vi "WriteFiles.vi"(8 "error in (no error)":errorcluster caption="错误输入（无错误）", 11 "EPUB 输入":refnum<class "EPUB.lvclass">) -> (0 "error out":errorcluster caption="错误输出", 3 "EPUB 输出":refnum<class "EPUB.lvclass">)   [LabVIEW 2016, in "EPUB.lvclass"]
uses:
  EPUB.lvclass
  EPUB.lvclass/EPUB.ctl
  <vilib>/NUAA/UTF8Convert.llb/Text2UTF8.vi
  <vilib>/Utility/libraryn.llb/Get File Extension.vi
  <userlib>/_OpenG.lib/string/string.llb/1D Array to String__ogtk.vi
  IMGSettings.vi
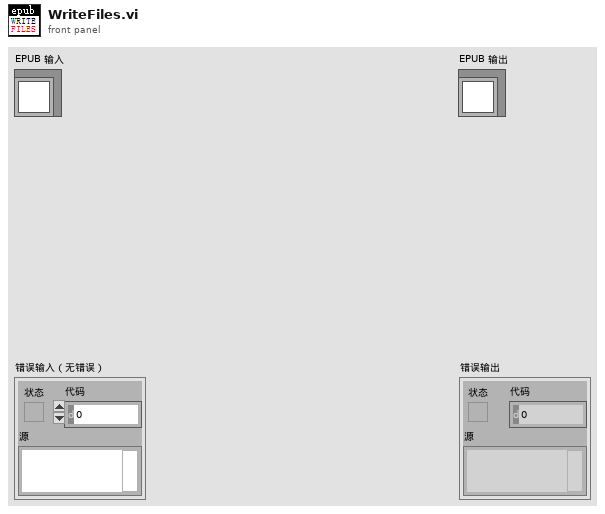
[diagram p1: front panel]
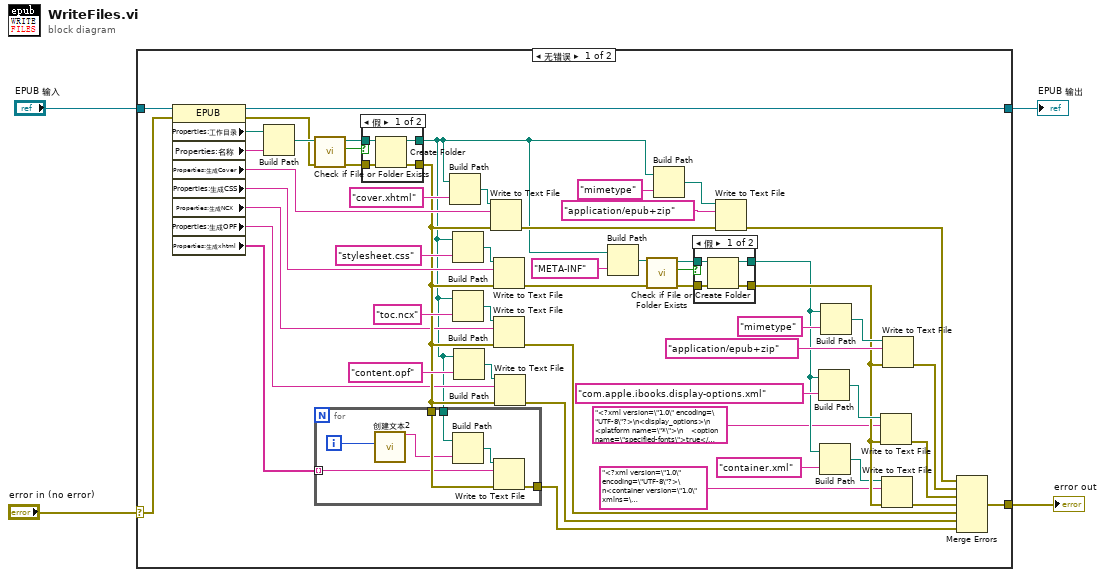
[diagram p0: block diagram]
diagram:
  n1 = case shown="无错误" "error in (no error)" {
    selector: "error in (no error)" -> [w56 w79]
    tunnel: [w12 w79] -> w3
    tunnel: [w57 w78] -> w1
    tunnel: "EPUB 输入" -> [w58 w78]
    frame No Error {
      n2 = property class="EPUB"(reference=w58, error in=w56) -> (reference out=w57:refnum<class "EPUB.lvclass">, error out=w52:errorcluster, "Properties:工作目录"=w54:path, "Properties:名称"=w55:string, "Properties:生成Cover"=w47:string, "Properties:生成CSS"=w43:string, "Properties:生成NCX"=w37:string, "Properties:生成OPF"=w36:string, "Properties:生成xhtml"=w35:string[])
      n3 = Build Path(base path=w54, name or relative path=w55) -> (appended path=w53:path)
      n4 = call <vilib>:"Check if File or Folder Exists.vi"("error in (no error)"=w52, "path"=w53) -> ("error out"=w51:errorcluster, "file or folder exists?"=w49:bool, "dup path"=w50:path)  [unwired: 7 in]
      n5 = case shown="假" w49 {
        tunnel: w51 -> [w75 w77]
        tunnel: w50 -> [w74 w76]
        tunnel: [w73 w77] -> w38
        tunnel: [w72 w76] -> w24
        frame False {
          n6 = Create Folder(path (use dialog)=w74, error in=w75) -> (created path=w72:path, error out=w73:errorcluster)  [unwired: 1 in, 1 out]
        }
        frame True {
        }
      }
      n7 = for {
        tunnel: w38 -> [w70]
        tunnel: w24 -> [w69]
        tunnel: w35 -> [w68] mode=indexing
        tunnel: [w67] -> w9
        i -> [w65]
        n8 = call "创建文本2"("idx"=w65) -> ("Result"=w66:string)  [unwired: 13 in, 1 out]
        n9 = Build Path(base path=w69, name or relative path=w66) -> (appended path=w71:path)
        n10 = Write to Text File(file (use dialog)=w71, text=w68, error in=w70) -> (error out=w67:errorcluster)  [unwired: 1 in, 2 out]
      }
      n11 = Build Path(base path=w24, name or relative path="cover.xhtml" ("名称或相对路径")) -> (appended path=w48:path)
      n12 = Build Path(base path=w24, name or relative path="stylesheet.css" ("名称或相对路径")) -> (appended path=w45:path)
      n13 = Build Path(base path=w24, name or relative path="toc.ncx" ("名称或相对路径")) -> (appended path=w42:path)
      n14 = Build Path(base path=w24, name or relative path="content.opf" ("名称或相对路径")) -> (appended path=w40:path)
      n15 = Write to Text File(file (use dialog)=w48, text=w47, error in=w38) -> (error out=w33:errorcluster)  [unwired: 1 in, 2 out]
      n16 = Write to Text File(file (use dialog)=w45, text=w43, error in=w38) -> (error out=w26:errorcluster)  [unwired: 1 in, 2 out]
      n17 = Write to Text File(file (use dialog)=w42, text=w37, error in=w38) -> (error out=w11:errorcluster)  [unwired: 1 in, 2 out]
      n18 = Write to Text File(file (use dialog)=w40, text=w36, error in=w38) -> (error out=w10:errorcluster)  [unwired: 1 in, 2 out]
      n19 = Build Path(base path=w24, name or relative path="META-INF" ("名称或相对路径")) -> (appended path=w28:path)
      n20 = call <vilib>:"Check if File or Folder Exists.vi"("error in (no error)"=w26, "path"=w28) -> ("error out"=w31:errorcluster, "file or folder exists?"=w29:bool, "dup path"=w30:path)  [unwired: 7 in]
      n21 = Build Path(base path=w24, name or relative path="mimetype" ("名称或相对路径")) -> (appended path=w27:path)
      n22 = case shown="假" w29 {
        tunnel: w31 -> [w62 w64]
        tunnel: w30 -> [w61 w63]
        tunnel: [w60 w64] -> w18
        tunnel: [w59 w63] -> w15
        frame False {
          n23 = Create Folder(path (use dialog)=w61, error in=w62) -> (created path=w59:path, error out=w60:errorcluster)  [unwired: 1 in, 1 out]
        }
        frame True {
        }
      }
      n24 = Write to Text File(file (use dialog)=w27, text="application/epub+zip", error in=w33) -> (error out=w5:errorcluster)  [unwired: 1 in, 2 out]
      n25 = Build Path(base path=w15, name or relative path="com.apple.ibooks.display-options.xml" ("名称或相对路径")) -> (appended path=w20:path)
      n26 = Build Path(base path=w15, name or relative path="container.xml" ("名称或相对路径")) -> (appended path=w17:path)
      n27 = Build Path(base path=w15, name or relative path="mimetype" ("名称或相对路径")) -> (appended path=w21:path)
      n28 = Write to Text File(file (use dialog)=w20, text="<?xml version=\"1.0\" encoding=\"UTF-8\"?>\n<display_options>\n  <platform name=\"*\">\n    <option name=\"specified-fonts\">true</option>\n  </platform>\n</display_options>", error in=w18) -> (error out=w7:errorcluster)  [unwired: 1 in, 2 out]
      n29 = Write to Text File(file (use dialog)=w17, text="<?xml version=\"1.0\" encoding=\"UTF-8\"?>\n<container version=\"1.0\" xmlns=\"urn:oasis:names:tc:opendocument:xmlns:container\">\n  <rootfiles>\n    <rootfile full-path=\"content.opf\" media-type=\"application/oebps-package+xml\" />\n  </rootfiles>\n</container>", error in=w18) -> (error out=w8:errorcluster)  [unwired: 1 in, 2 out]
      n30 = Write to Text File(file (use dialog)=w21, text="application/epub+zip", error in=w18) -> (error out=w6:errorcluster)  [unwired: 1 in, 2 out]
      n31 = Merge Errors(w5, w6, w7, w8, w11, w10, w9) -> (w12:errorcluster)
    }
    frame Error {
    }
  }
  "error out" <- w3
  "EPUB 输出" <- w1
